vi "VPD Device Engine.vi"() -> ()   [LabVIEW 2020]
uses:
  VPD Controls/VPD Pixel format.ctl
  VPD Controls/VPD Binning XX.ctl
  VPD Controls/VPD Scan Direction.ctl
  VPD Controls/VPD TDI Stages.ctl
  VPD Controls/VPD Test Pattern.ctl
  VPD Controls/VPD Note Type.ctl
  VPD Controls/VPD Actions.ctl
  Desktop/Vision Point LabVIEW/KYFGLib_lv.lvlib
panel:
  in  "Live Preview":bool
  in  "Test Pattern":T1 items=["Off", "Grey Horizontal Ramp", "Grey Diagonal Ramp", "Grey Diagonal Ramp Moving"]
  in  "Reverse X":bool
  in  "TDI Stages":T2=256 items=["4"=4, "8"=8, "16"=16, "32"=32, "64"=64, "96"=96, "128"=128, "160"=160, "192"=192, "224"=224, "240"=240, "248"=248, "252"=252, "256"=256]
  in  "Scan Direction":T3 items=["Forward", "Reverse", "LineIn"]
  in  "Binning Vertical (Y)":T4 items=["X1"=1, "X2"=2, "X4"=4, "X8"=8]
  in  "Binning Horizontal (X)":T4 items=["X1"=1, "X2"=2, "X4"=4, "X8"=8]
  in  "Pixel format":T5 items=["Mono8"=257, "Mono10"=258, "Mono12"=259]
  in  "Acquisition Line Rate [Hz]":dbl
  in  "Height (Y)":i64
  in  "Quit":bool
  in  "ROI (X)":cluster{"Width":i64, "Offset":i64}
  out "Camera handle":u32
  out "Frame Grabbers":string[](array[string])
  out "Frame Grabber handle":u32=65536 caption="FG handle"
  in  "Note Name":string="VPD Engine"
  # "REVERSEX\nSCAN MODE (TDI vs AREA)"
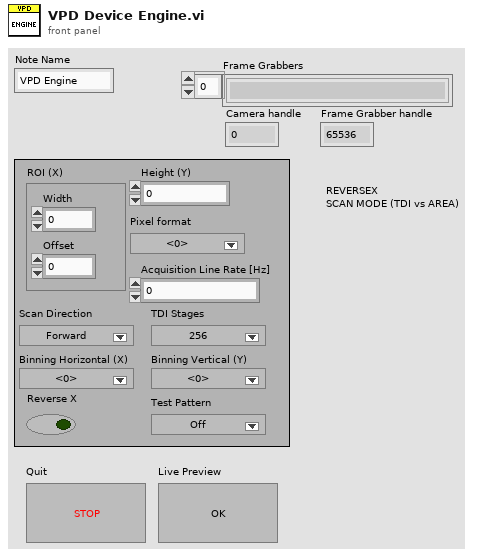
[diagram p1: front panel]
types:
  T1 = typedef "VPD Test Pattern.ctl" = u16
  T2 = typedef "VPD TDI Stages.ctl" = u16
  T3 = typedef "VPD Scan Direction.ctl" = u16
  T4 = typedef "VPD Binning XX.ctl" = u16
  T5 = typedef "VPD Pixel format.ctl" = i64
  T6 = typedef "VPD Note Type.ctl" = cluster{"TDI Actions":T7, "ROI (X)":i64[], "Cmd Received?":bool, "Height (Y)":i64, "Acquisition Line Rate":dbl, "Pixel format":T5, "Binning Horizontal (X)":T4, "Binning Vertical (Y)":T4, "Scan Direction":T3, "TDI Stages":T2, "Reverse X":bool, "Test Pattern":T1, "Live Preview":bool}
  T7 = typedef "VPD Actions.ctl" = enum16{"Nothing", "Set Height", "Set ROI", "Set Pixel format", "Set Line rate", "Set Binning Horizontal", "Set Binning Vertical", "Set Scan Direction", "Set TDI Stages", "Set Reverse X", "Set Test Pattern", "Live", "Quit"}
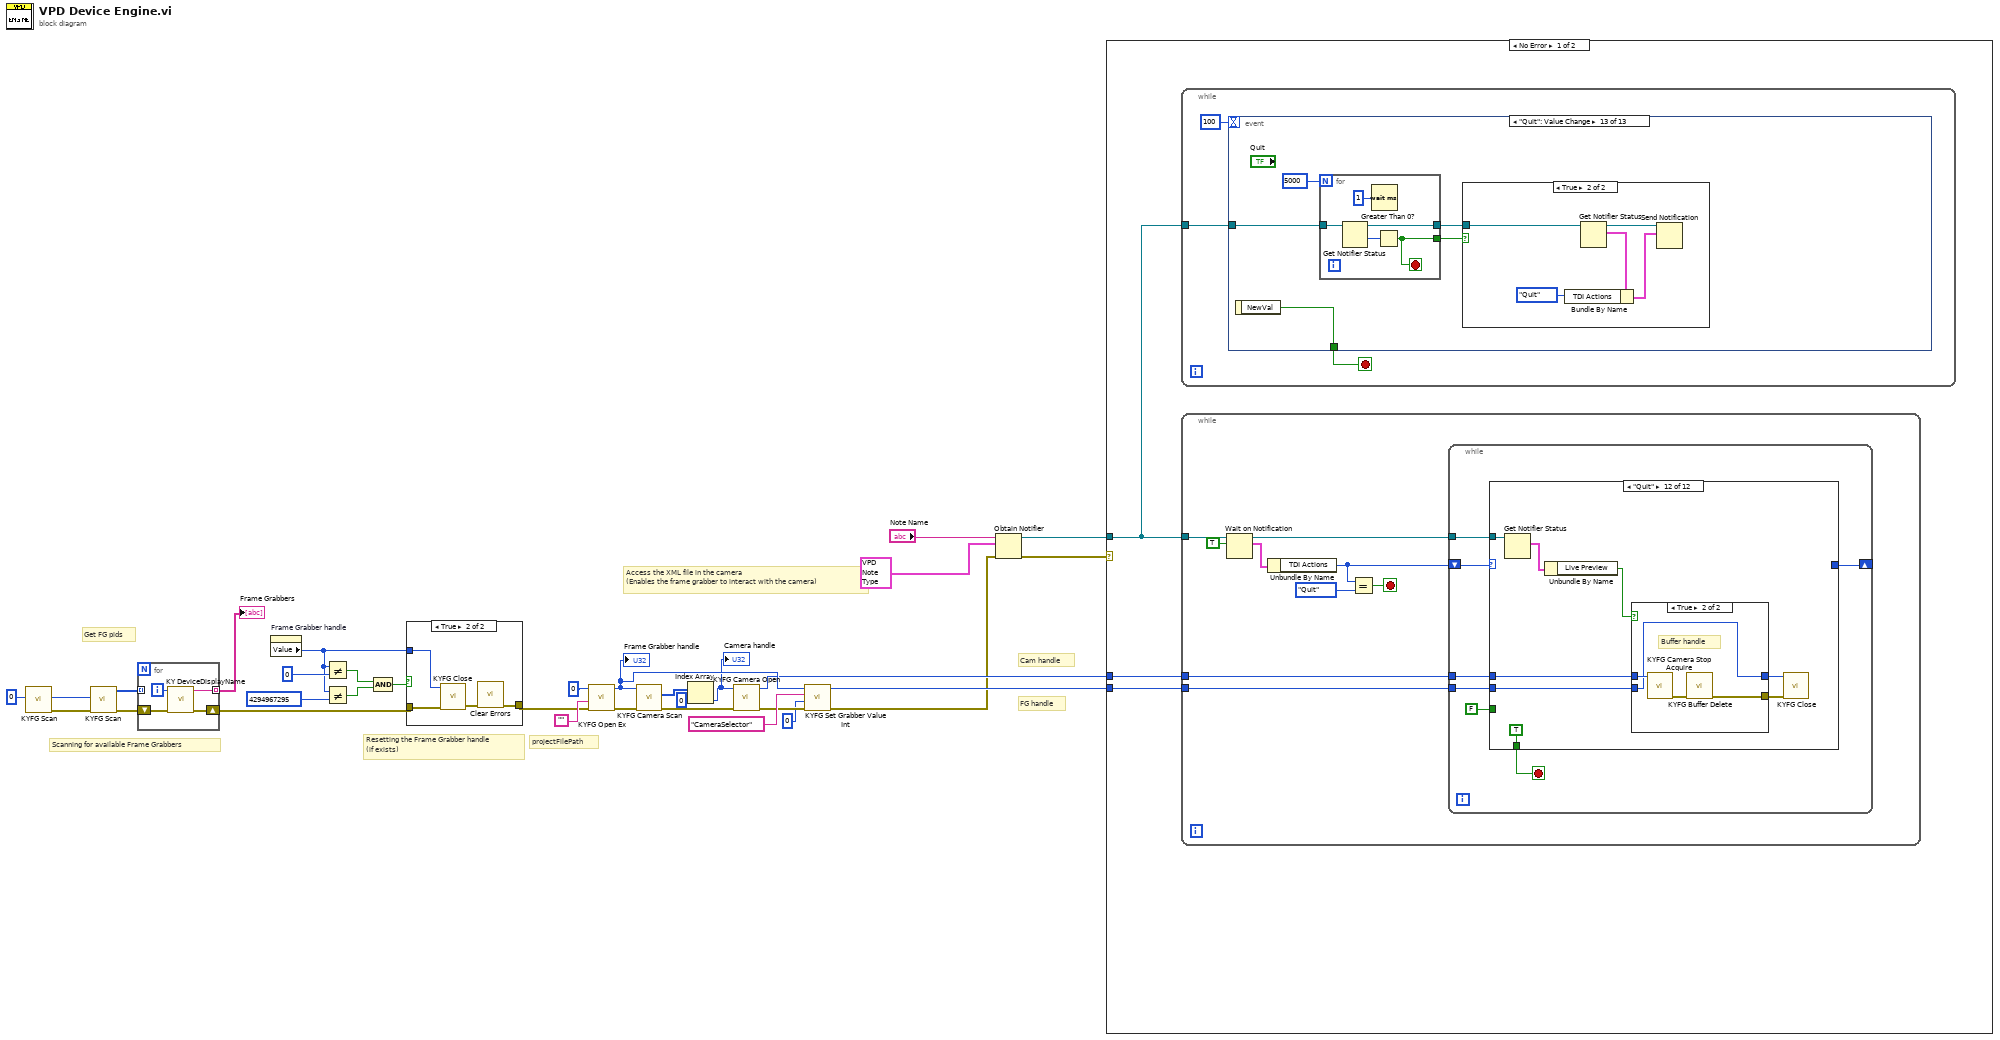
[diagram p0: block diagram]
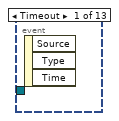
[diagram p2: hidden frame]
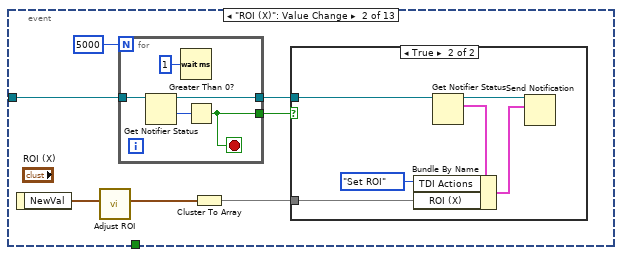
[diagram p3: hidden frame]
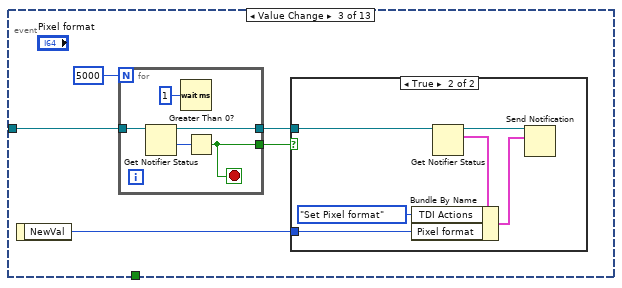
[diagram p5: hidden frame]
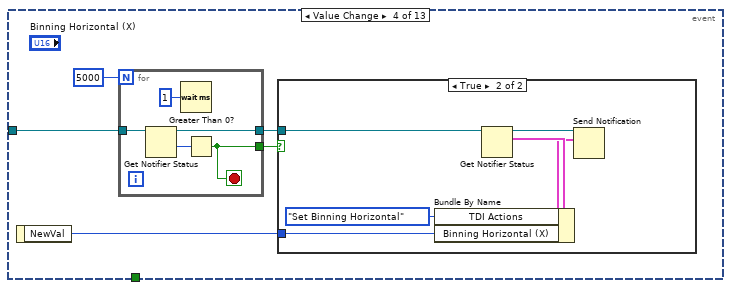
[diagram p7: hidden frame]
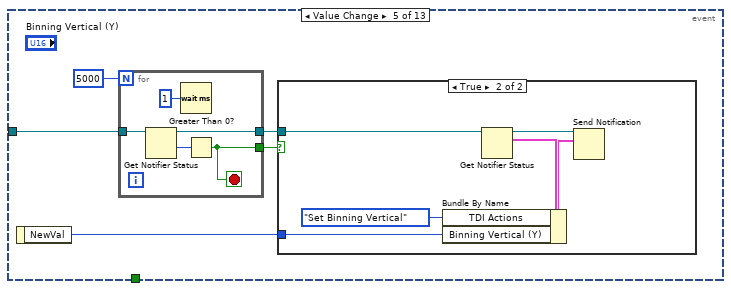
[diagram p9: hidden frame]
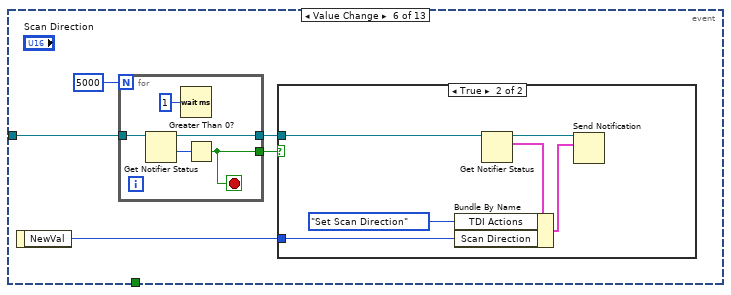
[diagram p11: hidden frame]
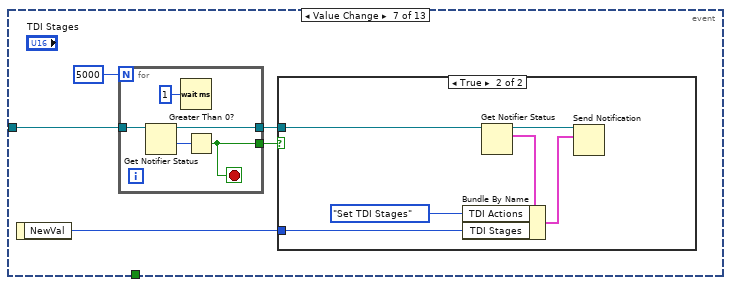
[diagram p13: hidden frame]
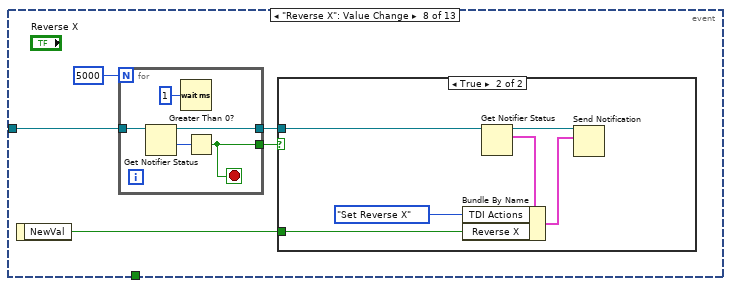
[diagram p15: hidden frame]
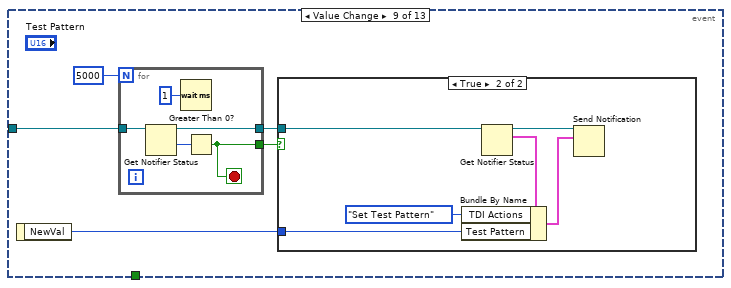
[diagram p17: hidden frame]
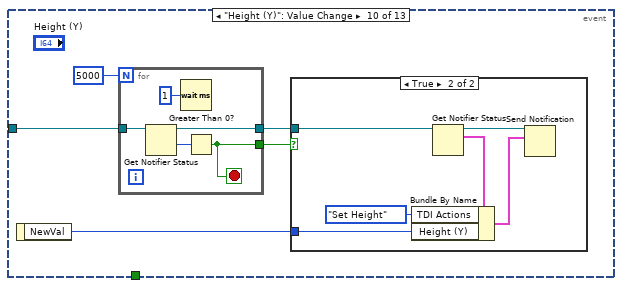
[diagram p19: hidden frame]
diagram:
  # "FG handle"
  # "Cam handle"
  # "Access the XML file in the camera\n(Enables the frame grabber to interact with the camera)"
  # "projectFilePath"
  # "Resetting the Frame Grabber handle\n(if exists)"
  # "Scanning for available Frame Grabbers"
  # "Get FG pids"
  n1 = call "KYFG Scan.vi"("count"=0) -> ("error out"=w20:errorcluster, "infosize"=w28:i32)  [unwired: 8 in, 1 out]
  n2 = call "KYFG Scan.vi"("error in (no error)"=w20, "count"=w28) -> ("error out"=w29:errorcluster, "pids_info"=w30:u32[])  [unwired: 7 in, 1 out]
  n3 = for {
    tunnel: w30 -> [_] mode=indexing
    shift-right: [w35] -> w16
    shift-left: w29 -> [w36]
    tunnel: [w33] -> w17 mode=indexing
    i -> [w34]
    n4 = call "KY DeviceDisplayName.vi"("error in (no error)"=w36, "index"=w34) -> ("error out"=w35:errorcluster, "function return"=w33:string)  [unwired: 8 in]
  }
  "Frame Grabbers" <- w17
  n5 = property on="Frame Grabber handle" class="DigNum (strict)"() -> ("Value"=w21:u32)  [unwired: 2 in, 2 out]
  n6 = Not Equal?(x=w21, y=u32 0) -> (x != y?=w27:bool)
  n7 = Not Equal?(x=w21, y=u32 4294967295) -> (x != y?=w26:bool)
  n8 = Compound Arithmetic op=AND(w27, w26) -> (w23:bool)
  n9 = case shown="True" w23 {
    tunnel: [w37 w39] -> w14
    tunnel: w21 -> [_ w41]
    tunnel: w16 -> [w37 w38]
    frame False {
    }
    frame True {
      n10 = call "KYFG Close.vi"("error in (no error)"=w38, "handle"=w41) -> ("error out"=w40:errorcluster)  [unwired: 8 in, 1 out]
      n11 = call <vilib>:"Clear Errors.vi"("error in (no error)"=w40) -> ("error out"=w39:errorcluster)  [unwired: 5 in, 1 out]
    }
  }
  n12 = call "KYFG Open Ex.vi"("error in (no error)"=w14, "projectFile"="", "index"=0) -> ("error out"=w19:errorcluster, "handle"=w8:u32)  [unwired: 7 in]
  "Frame Grabber handle" <- w8
  n13 = call "KYFG Camera Scan.vi"("error in (no error)"=w19, "handle"=w8) -> ("error out"=w10:errorcluster, "camHandleArray"=w13:u32[])  [unwired: 7 in, 1 out]
  n14 = Index Array(array=w13, index=0) -> (element=w6:u32)
  "Camera handle" <- w6
  n15 = call "KYFG Camera Open.vi"("error in (no error)"=w10, "camHandle"=w6) -> ("error out"=w9:errorcluster, "camHandle out"=w4:u32)  [unwired: 7 in, 1 out]
  n16 = call "KYFG Set Grabber Value Int.vi"("error in (no error)"=w9, "value"=i64 0, "paramName"="CameraSelector", "camHandle"=w8) -> ("error out"=w2:errorcluster, "camHandle out"=w3:u32)  [unwired: 6 in]
  n17 = Obtain Notifier(name (unnamed)="Note Name", notification data type=T6 {"TDI Actions"=enum."Set ROI", "ROI (X)"=[], "Cmd Received?"=FALSE, "Height (Y)"=0, "Acquisition Line Rate"=0.0, "Pixel format"=257, "Binning Horizontal (X)"=0, "Binning Vertical (Y)"=0, "Scan Direction"=0, "TDI Stages"=256, "Reverse X"=FALSE, "Test Pattern"=0, "Live Preview"=FALSE} ("TDI Note Type"), error in (no error)=w2) -> (notifier out=w31:refnum<notifier>, error out=w5:errorcluster)  [unwired: 1 in, 1 out]
  n18 = case shown="No Error" w5 {
    tunnel: w31 -> [w43 _]
    tunnel: w3 -> [w44 _]
    tunnel: w4 -> [w42 _]
    frame No Error {
      n19 = while {
        tunnel: w43 -> [w47]
        stop <- w45 stop-if-true
        n20 = event shown="[12] \"Quit\": Value Change" {
          selector: _ -> [_ _ _ _ _ _ _ _ _ _ _ _ _]
          dyn-events: _ -> [_ _ _ _ _ _ _ _ _ _ _ _ _]
          timeout: 100 -> [_ _ _ _ _ _ _ _ _ _ _ _ _]
          tunnel: w47 -> [_ w54 w69 w85 w101 w117 w133 w149 w165 w181 w197 w213 w232]
          tunnel: [_ _ _ _ _ _ _ _ _ _ _ _ w228] -> w45
          event Timeout {
            n21 = event-data() -> ()  [unwired: 1 in, 3 out]
          }
          event "ROI (X)": Value Change {
            n22 = event-data() -> ("NewVal"=w50:cluster{"Width":i64, "Offset":i64})  [unwired: 1 in]
            n23 = call "Adjust ROI.vi"("Horizontal Pixel ROI IN"=w50) -> ("Horizontal Pixel ROI OUT"=w49:cluster{i64, i64})  [unwired: 10 in]
            n24 = for {
              N: 5000 -> [_]
              tunnel: w54 -> [w65]
              tunnel: [w62] -> w52
              tunnel: [w61] -> w51
              stop <- w62 stop-if-true
              n25 = Get Notifier Status(notifier=w65) -> (notifier out=w61:refnum<notifier>, # waiting=w64:i32)  [unwired: 1 in, 3 out]
              n26 = Wait (ms)(milliseconds to wait=u32 1) -> ()  [unwired: 1 out]
              n27 = Greater Than 0?(x=w64) -> (x > 0?=w62:bool)
            }
            n28 = Cluster To Array(cluster=w49) -> (array=w48:i64[])
            n29 = case shown="True" w52 {
              tunnel: w51 -> [_ w56]
              tunnel: w48 -> [_ w55]
              frame False {
              }
              frame True {
                n30 = Get Notifier Status(notifier=w56) -> (notifier out=w58:refnum<notifier>, current notification=w60:T6)  [unwired: 1 in, 3 out]
                n31 = Bundle By Name(cluster=w60, "TDI Actions"=VPD_Actions."Set ROI", "ROI (X)"=w55) -> (w59:T6)
                n32 = Send Notification(notification=w59, notifier=w58) -> ()  [unwired: 1 in, 2 out]
              }
            }
          }
          event Value Change {
            n33 = event-data() -> ("NewVal"=w66:T5)  [unwired: 1 in]
            n34 = for {
              N: 5000 -> [_]
              tunnel: w69 -> [w81]
              tunnel: [w78] -> w67
              tunnel: [w77] -> w68
              stop <- w78 stop-if-true
              n35 = Get Notifier Status(notifier=w81) -> (notifier out=w77:refnum<notifier>, # waiting=w80:i32)  [unwired: 1 in, 3 out]
              n36 = Wait (ms)(milliseconds to wait=u32 1) -> ()  [unwired: 1 out]
              n37 = Greater Than 0?(x=w80) -> (x > 0?=w78:bool)
            }
            n38 = case shown="True" w67 {
              tunnel: w68 -> [_ w73]
              tunnel: w66 -> [_ w71]
              frame False {
              }
              frame True {
                n39 = Get Notifier Status(notifier=w73) -> (notifier out=w74:refnum<notifier>, current notification=w76:T6)  [unwired: 1 in, 3 out]
                n40 = Bundle By Name(cluster=w76, "TDI Actions"=VPD_Actions."Set Pixel format", "Pixel format"=w71) -> (w75:T6)
                n41 = Send Notification(notification=w75, notifier=w74) -> ()  [unwired: 1 in, 2 out]
              }
            }
          }
          event Value Change {
            n42 = event-data() -> ("NewVal"=w82:T4)  [unwired: 1 in]
            n43 = for {
              N: 5000 -> [_]
              tunnel: w85 -> [w97]
              tunnel: [w94] -> w83
              tunnel: [w93] -> w84
              stop <- w94 stop-if-true
              n44 = Get Notifier Status(notifier=w97) -> (notifier out=w93:refnum<notifier>, # waiting=w96:i32)  [unwired: 1 in, 3 out]
              n45 = Wait (ms)(milliseconds to wait=u32 1) -> ()  [unwired: 1 out]
              n46 = Greater Than 0?(x=w96) -> (x > 0?=w94:bool)
            }
            n47 = case shown="True" w83 {
              tunnel: w84 -> [_ w89]
              tunnel: w82 -> [_ w87]
              frame False {
              }
              frame True {
                n48 = Get Notifier Status(notifier=w89) -> (notifier out=w90:refnum<notifier>, current notification=w92:T6)  [unwired: 1 in, 3 out]
                n49 = Bundle By Name(cluster=w92, "TDI Actions"=VPD_Actions."Set Binning Horizontal", "Binning Horizontal (X)"=w87) -> (w91:T6)
                n50 = Send Notification(notification=w91, notifier=w90) -> ()  [unwired: 1 in, 2 out]
              }
            }
          }
          event Value Change {
            n51 = event-data() -> ("NewVal"=w98:T4)  [unwired: 1 in]
            n52 = for {
              N: 5000 -> [_]
              tunnel: w101 -> [w113]
              tunnel: [w110] -> w99
              tunnel: [w109] -> w100
              stop <- w110 stop-if-true
              n53 = Get Notifier Status(notifier=w113) -> (notifier out=w109:refnum<notifier>, # waiting=w112:i32)  [unwired: 1 in, 3 out]
              n54 = Wait (ms)(milliseconds to wait=u32 1) -> ()  [unwired: 1 out]
              n55 = Greater Than 0?(x=w112) -> (x > 0?=w110:bool)
            }
            n56 = case shown="True" w99 {
              tunnel: w100 -> [_ w105]
              tunnel: w98 -> [_ w103]
              frame False {
              }
              frame True {
                n57 = Get Notifier Status(notifier=w105) -> (notifier out=w106:refnum<notifier>, current notification=w108:T6)  [unwired: 1 in, 3 out]
                n58 = Bundle By Name(cluster=w108, "TDI Actions"=VPD_Actions."Set Binning Vertical", "Binning Vertical (Y)"=w103) -> (w107:T6)
                n59 = Send Notification(notification=w107, notifier=w106) -> ()  [unwired: 1 in, 2 out]
              }
            }
          }
          event Value Change {
            n60 = event-data() -> ("NewVal"=w114:T3)  [unwired: 1 in]
            n61 = for {
              N: 5000 -> [_]
              tunnel: w117 -> [w129]
              tunnel: [w126] -> w115
              tunnel: [w125] -> w116
              stop <- w126 stop-if-true
              n62 = Get Notifier Status(notifier=w129) -> (notifier out=w125:refnum<notifier>, # waiting=w128:i32)  [unwired: 1 in, 3 out]
              n63 = Wait (ms)(milliseconds to wait=u32 1) -> ()  [unwired: 1 out]
              n64 = Greater Than 0?(x=w128) -> (x > 0?=w126:bool)
            }
            n65 = case shown="True" w115 {
              tunnel: w116 -> [_ w121]
              tunnel: w114 -> [_ w119]
              frame False {
              }
              frame True {
                n66 = Get Notifier Status(notifier=w121) -> (notifier out=w122:refnum<notifier>, current notification=w124:T6)  [unwired: 1 in, 3 out]
                n67 = Bundle By Name(cluster=w124, "TDI Actions"=VPD_Actions."Set Scan Direction", "Scan Direction"=w119) -> (w123:T6)
                n68 = Send Notification(notification=w123, notifier=w122) -> ()  [unwired: 1 in, 2 out]
              }
            }
          }
          event Value Change {
            n69 = event-data() -> ("NewVal"=w130:T2)  [unwired: 1 in]
            n70 = for {
              N: 5000 -> [_]
              tunnel: w133 -> [w145]
              tunnel: [w142] -> w131
              tunnel: [w141] -> w132
              stop <- w142 stop-if-true
              n71 = Get Notifier Status(notifier=w145) -> (notifier out=w141:refnum<notifier>, # waiting=w144:i32)  [unwired: 1 in, 3 out]
              n72 = Wait (ms)(milliseconds to wait=u32 1) -> ()  [unwired: 1 out]
              n73 = Greater Than 0?(x=w144) -> (x > 0?=w142:bool)
            }
            n74 = case shown="True" w131 {
              tunnel: w132 -> [_ w137]
              tunnel: w130 -> [_ w135]
              frame False {
              }
              frame True {
                n75 = Get Notifier Status(notifier=w137) -> (notifier out=w138:refnum<notifier>, current notification=w140:T6)  [unwired: 1 in, 3 out]
                n76 = Bundle By Name(cluster=w140, "TDI Actions"=VPD_Actions."Set TDI Stages", "TDI Stages"=w135) -> (w139:T6)
                n77 = Send Notification(notification=w139, notifier=w138) -> ()  [unwired: 1 in, 2 out]
              }
            }
          }
          event "Reverse X": Value Change {
            n78 = event-data() -> ("NewVal"=w146:bool)  [unwired: 1 in]
            n79 = for {
              N: 5000 -> [_]
              tunnel: w149 -> [w161]
              tunnel: [w158] -> w147
              tunnel: [w157] -> w148
              stop <- w158 stop-if-true
              n80 = Get Notifier Status(notifier=w161) -> (notifier out=w157:refnum<notifier>, # waiting=w160:i32)  [unwired: 1 in, 3 out]
              n81 = Wait (ms)(milliseconds to wait=u32 1) -> ()  [unwired: 1 out]
              n82 = Greater Than 0?(x=w160) -> (x > 0?=w158:bool)
            }
            n83 = case shown="True" w147 {
              tunnel: w148 -> [_ w153]
              tunnel: w146 -> [_ w151]
              frame False {
              }
              frame True {
                n84 = Get Notifier Status(notifier=w153) -> (notifier out=w154:refnum<notifier>, current notification=w156:T6)  [unwired: 1 in, 3 out]
                n85 = Bundle By Name(cluster=w156, "TDI Actions"=VPD_Actions."Set Reverse X", "Reverse X"=w151) -> (w155:T6)
                n86 = Send Notification(notification=w155, notifier=w154) -> ()  [unwired: 1 in, 2 out]
              }
            }
          }
          event Value Change {
            n87 = event-data() -> ("NewVal"=w162:T1)  [unwired: 1 in]
            n88 = for {
              N: 5000 -> [_]
              tunnel: w165 -> [w177]
              tunnel: [w174] -> w163
              tunnel: [w173] -> w164
              stop <- w174 stop-if-true
              n89 = Get Notifier Status(notifier=w177) -> (notifier out=w173:refnum<notifier>, # waiting=w176:i32)  [unwired: 1 in, 3 out]
              n90 = Wait (ms)(milliseconds to wait=u32 1) -> ()  [unwired: 1 out]
              n91 = Greater Than 0?(x=w176) -> (x > 0?=w174:bool)
            }
            n92 = case shown="True" w163 {
              tunnel: w164 -> [_ w169]
              tunnel: w162 -> [_ w168]
              frame False {
              }
              frame True {
                n93 = Get Notifier Status(notifier=w169) -> (notifier out=w170:refnum<notifier>, current notification=w172:T6)  [unwired: 1 in, 3 out]
                n94 = Bundle By Name(cluster=w172, "TDI Actions"=VPD_Actions."Set Test Pattern", "Test Pattern"=w168) -> (w171:T6)
                n95 = Send Notification(notification=w171, notifier=w170) -> ()  [unwired: 1 in, 2 out]
              }
            }
          }
          event "Height (Y)": Value Change {
            n96 = event-data() -> ("NewVal"=w178:i64)  [unwired: 1 in]
            n97 = for {
              N: 5000 -> [_]
              tunnel: w181 -> [w193]
              tunnel: [w190] -> w179
              tunnel: [w189] -> w180
              stop <- w190 stop-if-true
              n98 = Get Notifier Status(notifier=w193) -> (notifier out=w189:refnum<notifier>, # waiting=w192:i32)  [unwired: 1 in, 3 out]
              n99 = Wait (ms)(milliseconds to wait=u32 1) -> ()  [unwired: 1 out]
              n100 = Greater Than 0?(x=w192) -> (x > 0?=w190:bool)
            }
            n101 = case shown="True" w179 {
              tunnel: w180 -> [_ w185]
              tunnel: w178 -> [_ w183]
              frame False {
              }
              frame True {
                n102 = Get Notifier Status(notifier=w185) -> (notifier out=w186:refnum<notifier>, current notification=w188:T6)  [unwired: 1 in, 3 out]
                n103 = Bundle By Name(cluster=w188, "TDI Actions"=VPD_Actions."Set Height", "Height (Y)"=w183) -> (w187:T6)
                n104 = Send Notification(notification=w187, notifier=w186) -> ()  [unwired: 1 in, 2 out]
              }
            }
          }
          event "Live Preview": Value Change {
            n105 = event-data() -> ("NewVal"=w194:bool)  [unwired: 1 in]
            n106 = for {
              N: 5000 -> [_]
              tunnel: w197 -> [w209]
              tunnel: [w206] -> w195
              tunnel: [w205] -> w196
              stop <- w206 stop-if-true
              n107 = Get Notifier Status(notifier=w209) -> (notifier out=w205:refnum<notifier>, # waiting=w208:i32)  [unwired: 1 in, 3 out]
              n108 = Wait (ms)(milliseconds to wait=u32 1) -> ()  [unwired: 1 out]
              n109 = Greater Than 0?(x=w208) -> (x > 0?=w206:bool)
            }
            n110 = case shown="True" w195 {
              tunnel: w196 -> [_ w201]
              tunnel: w194 -> [_ w199]
              frame False {
              }
              frame True {
                n111 = Get Notifier Status(notifier=w201) -> (notifier out=w202:refnum<notifier>, current notification=w204:T6)  [unwired: 1 in, 3 out]
                n112 = Bundle By Name(cluster=w204, "TDI Actions"=VPD_Actions."Live", "Live Preview"=w199) -> (w203:T6)
                n113 = Send Notification(notification=w203, notifier=w202) -> ()  [unwired: 1 in, 2 out]
              }
            }
          }
          event "Acquisition Line Rate [Hz]": Value Change {
            n114 = event-data() -> ("NewVal"=w210:dbl)  [unwired: 1 in]
            n115 = for {
              N: 5000 -> [_]
              tunnel: w213 -> [w227]
              tunnel: [w224] -> w211
              tunnel: [w223] -> w212
              stop <- w224 stop-if-true
              n116 = Get Notifier Status(notifier=w227) -> (notifier out=w223:refnum<notifier>, # waiting=w226:i32)  [unwired: 1 in, 3 out]
              n117 = Wait (ms)(milliseconds to wait=u32 1) -> ()  [unwired: 1 out]
              n118 = Greater Than 0?(x=w226) -> (x > 0?=w224:bool)
            }
            n119 = case shown="False" w211 {
              tunnel: w212 -> [_ w220]
              tunnel: w210 -> [_ w217]
              frame False {
              }
              frame True {
                n120 = Get Notifier Status(notifier=w220) -> (notifier out=w221:refnum<notifier>, current notification=w218:T6)  [unwired: 1 in, 3 out]
                n121 = Unbundle By Name(w218) -> ("Pixel format"=w215:T5)
                n122 = call "Coerce Line Rate.vi"("Line rate IN"=w217, "Pixel format"=w215) -> ("Line rate OUT"=w216:dbl)  [unwired: 9 in]
                n123 = Bundle By Name(cluster=w218, "TDI Actions"=VPD_Actions."Set Line rate", "Acquisition Line Rate"=w216) -> (w222:T6)
                n124 = Send Notification(notification=w222, notifier=w221) -> ()  [unwired: 1 in, 2 out]
              }
            }
          }
          event "Quit": Value Change {
            n125 = event-data() -> ("NewVal"=w228:bool)  [unwired: 1 in]
            n126 = for {
              N: 5000 -> [_]
              tunnel: w232 -> [w242]
              tunnel: [w239] -> w230
              tunnel: [w238] -> w229
              stop <- w239 stop-if-true
              n127 = Get Notifier Status(notifier=w242) -> (notifier out=w238:refnum<notifier>, # waiting=w241:i32)  [unwired: 1 in, 3 out]
              n128 = Wait (ms)(milliseconds to wait=u32 1) -> ()  [unwired: 1 out]
              n129 = Greater Than 0?(x=w241) -> (x > 0?=w239:bool)
            }
            n130 = case shown="True" w230 {
              tunnel: w229 -> [_ w233]
              frame False {
              }
              frame True {
                n131 = Get Notifier Status(notifier=w233) -> (notifier out=w235:refnum<notifier>, current notification=w237:T6)  [unwired: 1 in, 3 out]
                n132 = Bundle By Name(cluster=w237, "TDI Actions"=VPD_Actions."Quit") -> (w236:T6)
                n133 = Send Notification(notification=w236, notifier=w235) -> ()  [unwired: 1 in, 2 out]
              }
            }
          }
        }
      }
      n134 = while {
        tunnel: w43 -> [w251]
        tunnel: w44 -> [w244]
        tunnel: w42 -> [w243]
        stop <- w247 stop-if-true
        n135 = Wait on Notification(notifier=w251, ignore previous (F)=TRUE) -> (notifier out=w246:refnum<notifier>, notification=w249:T6)  [unwired: 2 in, 2 out]
        n136 = Unbundle By Name(w249) -> ("TDI Actions"=w245:T7)
        n137 = Equal?(x=w245, y=VPD_Actions."Quit") -> (x = y?=w247:bool)
        n138 = while {
          tunnel: w246 -> [w254]
          shift-right: [w255] -> _
          shift-left: w245 -> [w258]
          tunnel: w244 -> [w253]
          tunnel: w243 -> [w252]
          stop <- w256 stop-if-true
          n139 = case shown="\"Quit\"" w258 {
            tunnel: FALSE -> [_ w269 w278 w287 w296 w305 w314 w323 w332 w339 w346 _]
            tunnel: [_ w269 w278 w287 w296 w305 w314 w323 w332 w339 w346 TRUE] -> w256
            tunnel: [_ VPD_Actions."Nothing" ("y") VPD_Actions."Nothing" ("y") VPD_Actions."Nothing" ("y") VPD_Actions."Nothing" ("y") VPD_Actions."Nothing" ("y") VPD_Actions."Nothing" ("y") VPD_Actions."Nothing" ("y") VPD_Actions."Nothing" ("y") VPD_Actions."Nothing" ("y") VPD_Actions."Nothing" ("y") _] -> w255
            tunnel: w254 -> [_ w268 w277 w286 w295 w304 w313 w322 w331 w338 w343 w352]
            tunnel: w253 -> [_ _ _ _ _ _ _ _ _ _ w340 w348]
            tunnel: w252 -> [_ w260 w274 w283 w292 w301 w310 w319 w328 w335 _ w350]
            frame "Nothing", Default {
            }
            frame "Set ROI" {
              n140 = Get Notifier Status(notifier=w268) -> (current notification=w267:T6)  [unwired: 1 in, 4 out]
              n141 = Unbundle By Name(w267) -> ("ROI (X)"=w263:i64[])
              n142 = Index Array(array=w263) -> (element #1=w261:i64, element #2=w262:i64)  [unwired: 2 in]
              n143 = call "KYFG Set Camera Value.vi"("paramValue"=w262, "paramName"="OffsetX", "camHandle"=w260) -> ("camHandle out"=w265:u32)  [unwired: 7 in, 1 out]
              n144 = call "KYFG Set Camera Value.vi"("paramValue"=w261, "paramName"="Width", "camHandle"=w265) -> ()  [unwired: 7 in, 2 out]
            }
            frame "Set Pixel format" {
              n145 = Get Notifier Status(notifier=w277) -> (current notification=w276:T6)  [unwired: 1 in, 4 out]
              n146 = Unbundle By Name(w276) -> ("Pixel format"=w272:T5)
              n147 = Type Cast(type=i64 0, x=w272) -> (*(type *) &x=w270:i64)
              n148 = call "KYFG Set Camera Value.vi"("paramValue"=w270, "paramName"="PixelFormat", "camHandle"=w274) -> ()  [unwired: 7 in, 2 out]
            }
            frame "Set Binning Horizontal" {
              n149 = Get Notifier Status(notifier=w286) -> (current notification=w285:T6)  [unwired: 1 in, 4 out]
              n150 = Unbundle By Name(w285) -> ("Binning Horizontal (X)"=w281:T4)
              n151 = Type Cast(type=i64 0, x=w281) -> (*(type *) &x=w279:i64)
              n152 = call "KYFG Set Camera Value.vi"("paramValue"=w279, "paramName"="BinningHorizontal", "camHandle"=w283) -> ()  [unwired: 7 in, 2 out]
            }
            frame "Set Binning Vertical" {
              n153 = Get Notifier Status(notifier=w295) -> (current notification=w294:T6)  [unwired: 1 in, 4 out]
              n154 = Unbundle By Name(w294) -> ("Binning Vertical (Y)"=w290:T4)
              n155 = Type Cast(type=i64 0, x=w290) -> (*(type *) &x=w288:i64)
              n156 = call "KYFG Set Camera Value.vi"("paramValue"=w288, "paramName"="BinningVertical", "camHandle"=w292) -> ()  [unwired: 7 in, 2 out]
            }
            frame "Set Scan Direction" {
              n157 = Get Notifier Status(notifier=w304) -> (current notification=w303:T6)  [unwired: 1 in, 4 out]
              n158 = Unbundle By Name(w303) -> ("Scan Direction"=w299:T3)
              n159 = Type Cast(type=i64 0, x=w299) -> (*(type *) &x=w297:i64)
              n160 = call "KYFG Set Camera Value.vi"("paramValue"=w297, "paramName"="ScanDirection", "camHandle"=w301) -> ()  [unwired: 7 in, 2 out]
            }
            frame "Set TDI Stages" {
              n161 = Get Notifier Status(notifier=w313) -> (current notification=w312:T6)  [unwired: 1 in, 4 out]
              n162 = Unbundle By Name(w312) -> ("Scan Direction"=w308:T3)
              n163 = Type Cast(type=i64 0, x=w308) -> (*(type *) &x=w306:i64)
              n164 = call "KYFG Set Camera Value.vi"("paramValue"=w306, "paramName"="TDIStagesP1", "camHandle"=w310) -> ()  [unwired: 7 in, 2 out]
            }
            frame "Set Reverse X" {
              n165 = Get Notifier Status(notifier=w322) -> (current notification=w321:T6)  [unwired: 1 in, 4 out]
              n166 = Unbundle By Name(w321) -> ("Reverse X"=w317:bool)
              n167 = Type Cast(type=i64 0, x=w317) -> (*(type *) &x=w315:i64)
              n168 = call "KYFG Set Camera Value.vi"("paramValue"=w315, "paramName"="ReverseX", "camHandle"=w319) -> ()  [unwired: 7 in, 2 out]
            }
            frame "Set Test Pattern" {
              n169 = Get Notifier Status(notifier=w331) -> (current notification=w330:T6)  [unwired: 1 in, 4 out]
              n170 = Unbundle By Name(w330) -> ("Test Pattern"=w326:T1)
              n171 = Type Cast(type=i64 0, x=w326) -> (*(type *) &x=w324:i64)
              n172 = call "KYFG Set Camera Value.vi"("paramValue"=w324, "paramName"="TestPattern", "camHandle"=w328) -> ()  [unwired: 7 in, 2 out]
            }
            frame "Set Line rate" {
              n173 = Get Notifier Status(notifier=w338) -> (current notification=w337:T6)  [unwired: 1 in, 4 out]
              n174 = Unbundle By Name(w337) -> ("Acquisition Line Rate"=w333:dbl)
              n175 = call "KYFG Set Camera Value Float.vi"("value"=w333, "paramName"="AcquisitionLineRate", "camHandle"=w335) -> ()  [unwired: 7 in, 2 out]
            }
            frame "Set Height" {
              n176 = Get Notifier Status(notifier=w343) -> (current notification=w344:T6)  [unwired: 1 in, 4 out]
              n177 = Unbundle By Name(w344) -> ("Height (Y)"=w342:i64)
              n178 = call "KYFG Set Grabber Value Int.vi"("value"=w342, "paramName"="SegmentsPerBuffer", "camHandle"=w340) -> ()  [unwired: 7 in, 2 out]
            }
            frame "Quit" {
              n179 = Get Notifier Status(notifier=w352) -> (current notification=w353:T6)  [unwired: 1 in, 4 out]
              n180 = Unbundle By Name(w353) -> ("Live Preview"=w351:bool)
              n181 = case shown="True" w351 {
                tunnel: w350 -> [w356 w361]
                tunnel: [w357 w359] -> w349
                tunnel: w348 -> [w355 w358]
                tunnel: [w355 w358] -> w347
                frame False {
                  n182 = call "KYFG Camera Stop Acquire.vi"("camHandle"=w356) -> ("error out"=w357:errorcluster)  [unwired: 9 in, 1 out]
                }
                frame True {
                  # "Buffer handle"
                  n183 = call "KYFG Camera Stop Acquire.vi"("camHandle"=w361) -> ("error out"=w360:errorcluster)  [unwired: 9 in, 1 out]
                  n184 = call "KYFG Buffer Delete.vi"("error in (no error)"=w360) -> ("error out"=w359:errorcluster)  [unwired: 10 in]
                }
              }
              n185 = call "KYFG Close.vi"("error in (no error)"=w349, "handle"=w347) -> ()  [unwired: 8 in, 2 out]
            }
          }
        }
      }
    }
    frame Error {
    }
  }
